vi "WriteNumber.vi"(8 "error in (no error)":errorcluster, 10 "Numeric":dbl, 11 "Byte Stream File in":refnum<file>) -> (0 "error out":errorcluster, 3 "Byte Stream File out":refnum<file>)   [LabVIEW 2023]
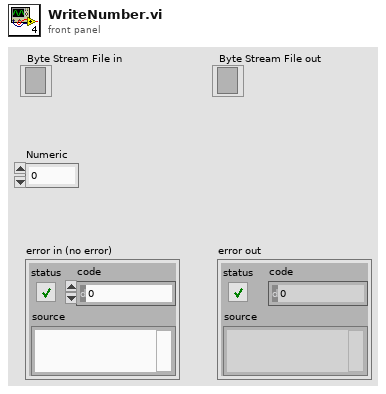
[diagram p1: front panel]
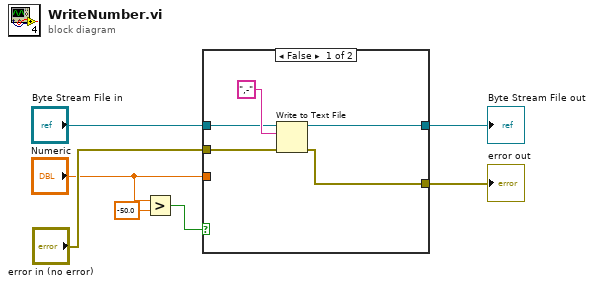
[diagram p0: block diagram]
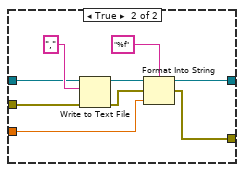
[diagram p2: hidden frame]
diagram:
  n1 = Greater?(x="Numeric", y=-50.0) -> (0:w1:bool)
  n2 = case shown="False" w1 {
    tunnel: "error in (no error)" -> [w9 w21]
    tunnel: [w8 w20] -> w6
    tunnel: "Numeric" -> [_ w15]
    tunnel: [w10 w14] -> w5
    tunnel: "Byte Stream File in" -> [w11 w13]
    frame False {
      n3 = Write to Text File(file (use dialog)=w11, text=",-", error in=w9) -> (refnum out=w10:refnum<file>, error out=w8:errorcluster)  [unwired: 1 in, 1 out]
    }
    frame True {
      n4 = Write to Text File(file (use dialog)=w13, text=",", error in=w21) -> (refnum out=w17:refnum<file>, error out=w18:errorcluster)  [unwired: 1 in, 1 out]
      n5 = Format Into String(format string="%f", initial string=w17, error in=w18, w15) -> (resulting string=w14:refnum<file>, error out=w20:errorcluster)
    }
  }
  "error out" <- w6
  "Byte Stream File out" <- w5
